vi "getDeviceType.vi"(11 "Device in":string) -> (3 "devicetype":string)   [LabVIEW 2020]
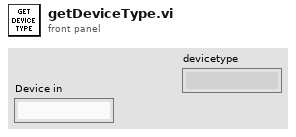
[diagram p1: front panel]
types:
  T1 = typedef "mysql_authentication.ctl" = cluster{"User":string, "Password":string, "Database":string}
  T2 = cluster{"Port":u16, "IP Address":string, "Authentication":T1}
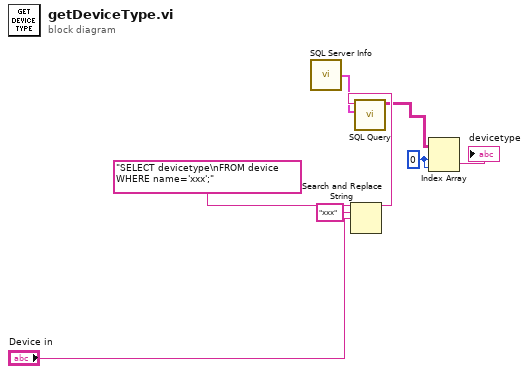
[diagram p0: block diagram]
diagram:
  w2 = 0 ("index (row)")
  n1 = call "SQL Server Info.vi"() -> ("SQL Server Info"=w4:T2)
  n2 = Search and Replace String(input string="SELECT devicetype\nFROM device WHERE name='xxx';", search string="xxx", replace string="Device in") -> (result string=w8:string)  [unwired: 5 in, 3 out]
  n3 = call "SQL Query.vi"("SQL Server Info"=w4, "Query"=w8) -> ("data"=w3:string[][])  [unwired: 8 in, 1 out]
  n4 = Index Array(array=w3, index (row)=w2, index (col)=w2) -> (element=→"devicetype":string)
